vi "Ping Sensor.vi"(8 "error in":errorcluster) -> (0 "error out":errorcluster)   [LabVIEW 2016, in "Vision Server.lvclass"]
uses:
  Vision Server.lvclass
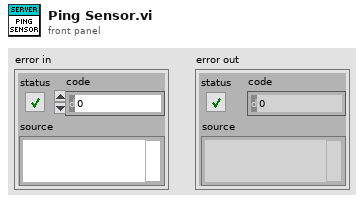
[diagram p1: front panel]
types:
  T1 = typedef "Vision Server.lvclass/Message Type.ctl" = cluster{"type":string, "message":string}
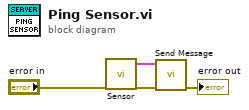
[diagram p0: block diagram]
diagram:
  n1 = call "Sensor.vi"() -> ("camera mode vision"=w1:T1)  [unwired: 2 in]
  n2 = call "Send Message.vi"("error in"="error in", "Message"=w1) -> ("error out"=→"error out":errorcluster)  [unwired: 9 in]
